vi "fetch_image.vi"(8 "error in (no error)":errorcluster, 11 "DL090216Display in":refnum<class "DisplayDL090216.lvclass">) -> (0 "error out":errorcluster, 1 "channels array empty?":bool, 2 "image (channels)":refnum<class "Image.lvclass">[](array[class]), 3 "DL090216Display out":refnum<class "DisplayDL090216.lvclass">, 4 "# elements in queue":i32, 6 "finished?":bool[](array[boolean]))   [LabVIEW 2010, in "DisplayDL090216.lvclass"]
uses:
  DisplayDL090216.lvclass
  common/classes/Image/Image/Image.lvclass
  GenericDisplay/GenericDisplay/GenericDisplay.lvclass
  DisplayDL090216.lvclass/DisplayDL090216.ctl
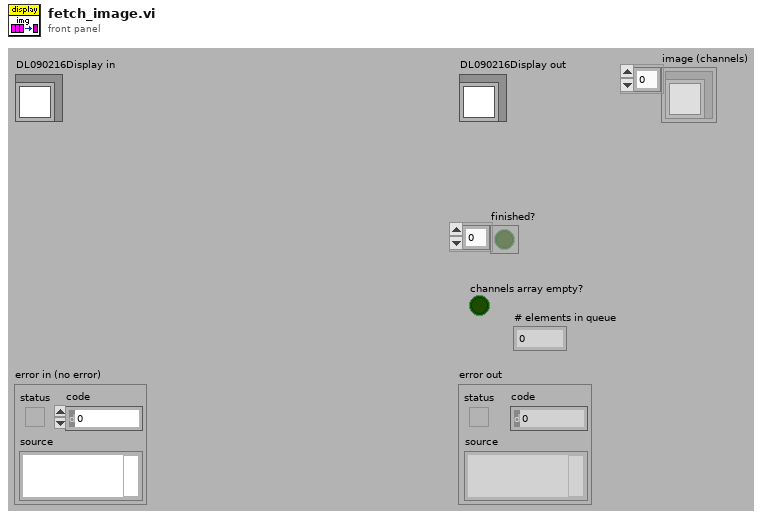
[diagram p1: front panel]
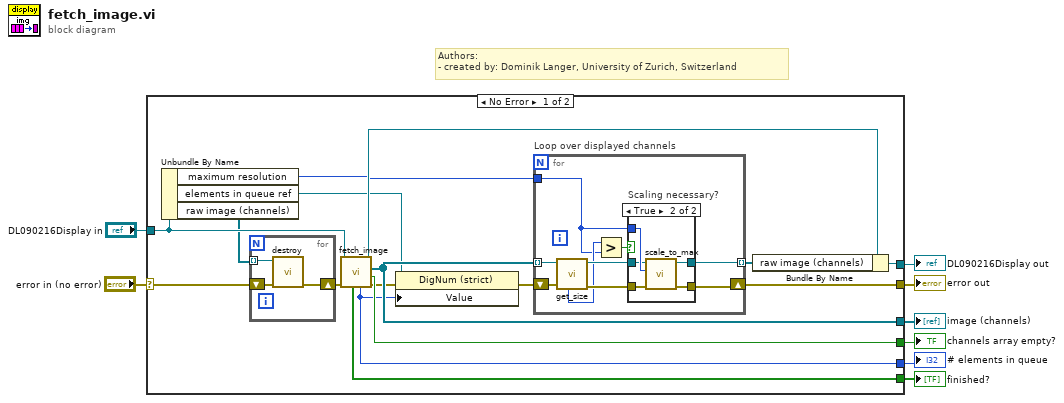
[diagram p0: block diagram]
diagram:
  # "Authors: \n- created by: Dominik Langer, University of Zurich, Switzerland"
  n1 = case shown="No Error" "error in (no error)" {
    selector: "error in (no error)" -> [w22 w45]
    tunnel: [w13 w45] -> w7
    tunnel: [w24 w44] -> w5
    tunnel: "DL090216Display in" -> [w20 w44]
    tunnel: [w15 _] -> w2
    tunnel: [w14 _] -> w4
    tunnel: [w16 _] -> w3
    tunnel: [w9 _] -> w1
    frame No Error {
      n2 = Unbundle By Name(w20) -> ("maximum resolution"=w18:i32, "elements in queue ref"=w12:refnum<vi>, "raw image (channels)"=w19:refnum<class "Image.lvclass">[])
      n3 = for {
        shift-right: [w41] -> w21
        shift-left: w22 -> [w43]
        tunnel: w19 -> [w42] mode=indexing
        n4 = call-dynamic "destroy.vi"("error in (no error)"=w43, "Image in"=w42) -> ("error out"=w41:errorcluster)  [unwired: 9 out]
      }
      n5 = call-parent "fetch_image.vi"("error in (no error)"=w21, "GenericToplevelComponent in"=w20) -> ("error out"=w10:errorcluster, "channels array empty?"=w15:bool, "image (channels)"=w14:refnum<class "Image.lvclass">[], "GenericToplevelComponent out"=w23:refnum<class "DisplayDL090216.lvclass">, "# elements in queue"=w9:i32, "finished?"=w16:bool[])  [unwired: 4 out]
      n6 = property class="DigNum (strict)"(reference=w12, error in=w10, "Value"=w9) -> (error out=w11:errorcluster)  [unwired: 1 out]
      n7 = for "Loop over displayed channels" {
        tunnel: w14 -> [w25] mode=indexing
        shift-right: [w33] -> w13
        shift-left: w11 -> [w26]
        tunnel: [w32] -> w17 mode=indexing
        tunnel: w18 -> [w27]
        n8 = call-dynamic "get_size.vi"("error in (no error)"=w26, "Image in"=w25) -> ("error out"=w30:errorcluster, "Image out"=w31:refnum<class "Image.lvclass">, "max resolution"=w29:i32)  [unwired: 2 in, 5 out]
        n9 = Greater?(x=w29, y=w27) -> (0:w28:bool)
        n10 = case "Scaling necessary?" shown="True" w28 {
          tunnel: [w35 w37] -> w33
          tunnel: [w34 w36] -> w32
          tunnel: w27 -> [_ w40]
          tunnel: w31 -> [w34 w39]
          tunnel: w30 -> [w35 w38]
          frame False {
          }
          frame True {
            n11 = call-dynamic "scale_to_max.vi"("error in (no error)"=w38, "max length (pixels)"=w40, "Image in"=w39) -> ("error out"=w37:errorcluster, "Image out"=w36:refnum<class "Image.lvclass">)  [unwired: 7 in]
          }
        }
      }
      n12 = Bundle By Name(cluster=w23, "raw image (channels)"=w17) -> (w24:refnum<class "DisplayDL090216.lvclass">)
    }
    frame Error {
    }
  }
  "error out" <- w7
  "DL090216Display out" <- w5
  "image (channels)" <- w4
  "finished?" <- w3
  "channels array empty?" <- w2
  "# elements in queue" <- w1
